vi "ScriptedAutonomous.vi"   [LabVIEW 2015]
uses:
  Common Code/commandCluster.ctl
  Common Code/Change Detect Int.vi
  Robot Global Data.vi
types:
  T1 = typedef "commandCluster.ctl" = cluster{"Step ID":i16, "Command Type":i16, "Drive X":sgl, "Drive Y":sgl, "Heading":sgl, "Max Exec. Time":i16, "Jump Type":i32, "Jump To":i16, "Jump Condition":i16, "Async Drive?":i16, "Roller Mode":i16, "Roller Align":i16, "Roller Closed?":i16, "Wait Condition":i16, "Elevator Mode":i16, "Elevator Command":i16, "Roller State":i16, "Hold Low?":i16, "Num Totes":i16, "Num Cans":dbl, "Past Distance":dbl, "Store Can?":dbl, "X Speed":dbl, "Y Speed":dbl, "Yaw Angle Set":dbl, "Grab Can":dbl, "Roller Overide Speed":dbl, "Force Load?":sgl, "Set Idle":sgl, "Eject":sgl, "Pike Action":sgl, "Pivot Speed":dbl, "Height":dbl}
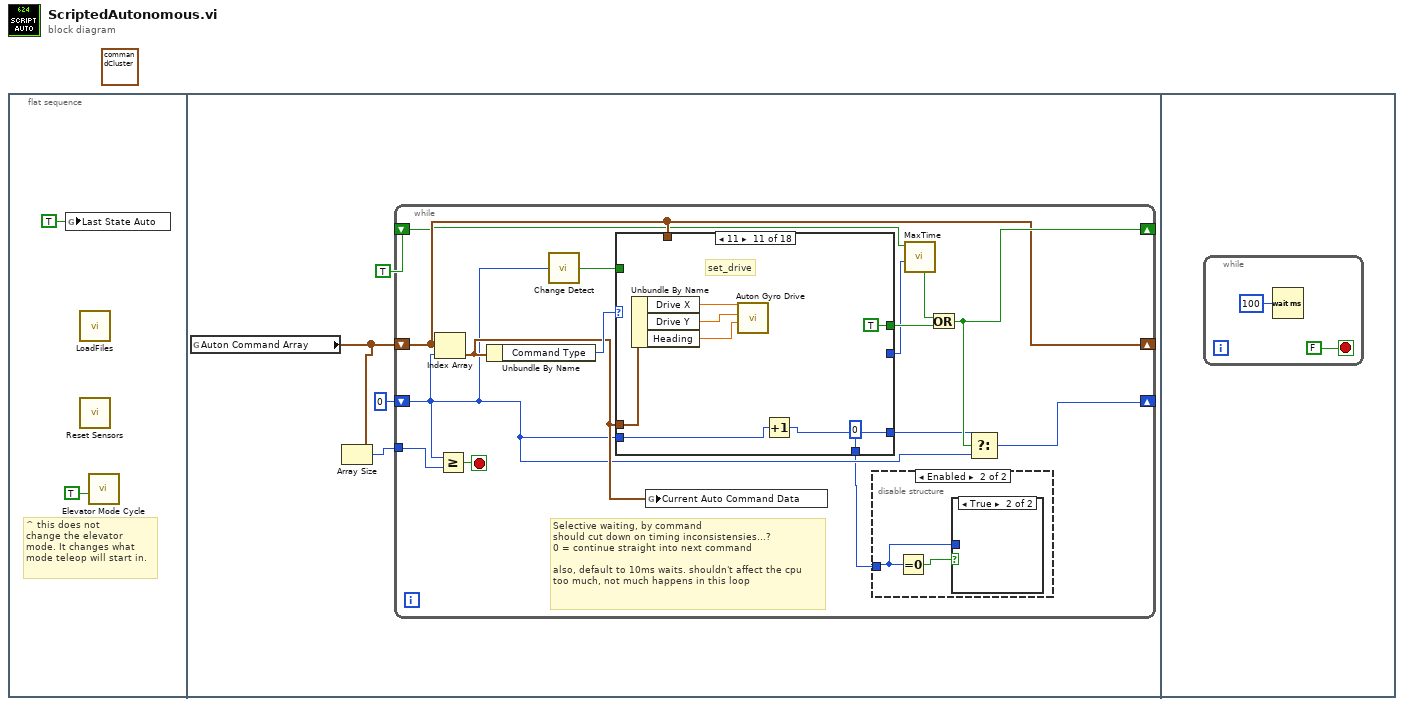
[diagram p0: block diagram]
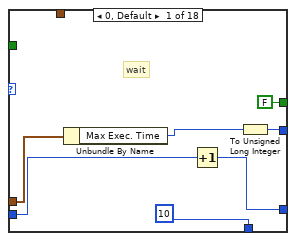
[diagram p2: hidden frame]
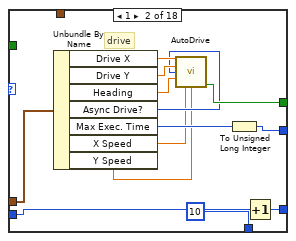
[diagram p3: hidden frame]
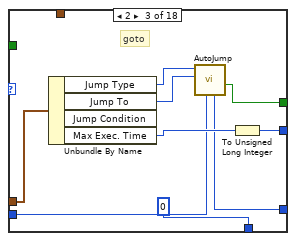
[diagram p4: hidden frame]
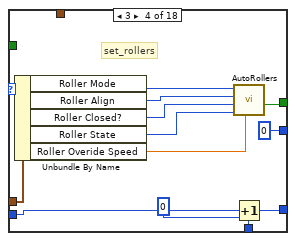
[diagram p5: hidden frame]
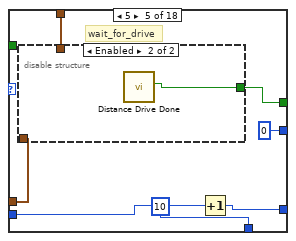
[diagram p6: hidden frame]
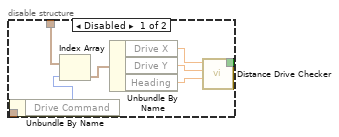
[diagram p7: hidden frame]
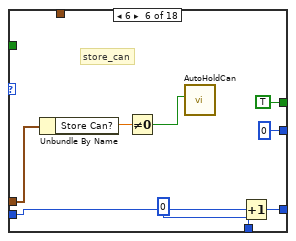
[diagram p8: hidden frame]
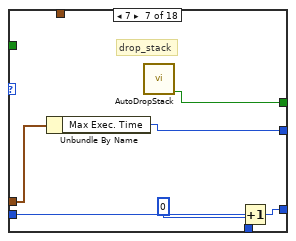
[diagram p9: hidden frame]
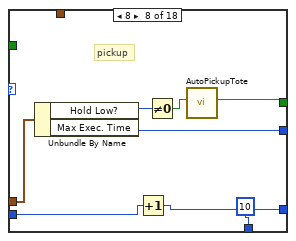
[diagram p10: hidden frame]
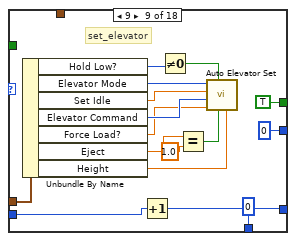
[diagram p11: hidden frame]
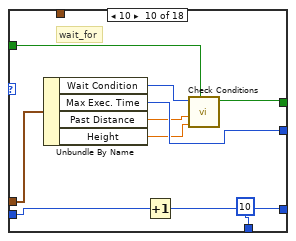
[diagram p12: hidden frame]
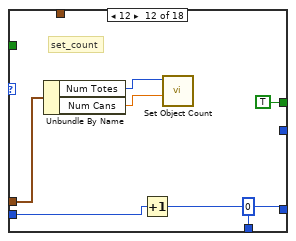
[diagram p13: hidden frame]
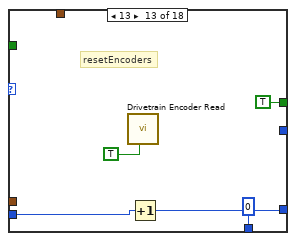
[diagram p14: hidden frame]
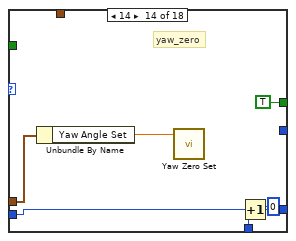
[diagram p15: hidden frame]
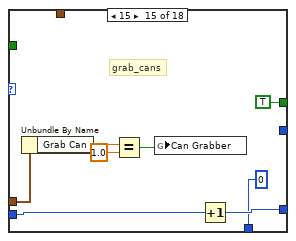
[diagram p16: hidden frame]
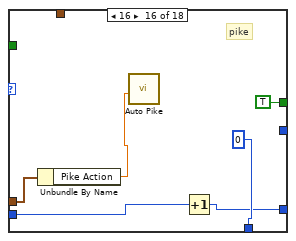
[diagram p17: hidden frame]
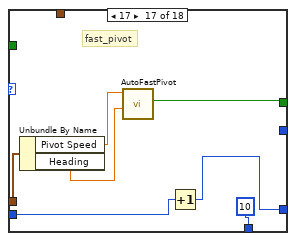
[diagram p18: hidden frame]
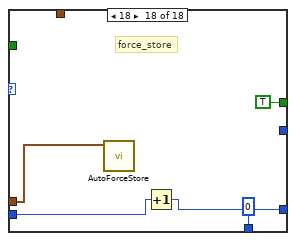
[diagram p19: hidden frame]
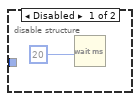
[diagram p20: hidden frame]
diagram:
  (unwired) T1 {"Step ID"=0, "Command Type"=0, "Drive X"=0.0, "Drive Y"=0.0, "Heading"=0.0, "Max Exec. Time"=0, "Jump Type"=0, "Jump To"=0, "Jump Condition"=0, "Async Drive?"=0, "Roller Mode"=0, "Roller Align"=0, "Roller Closed?"=0, "Wait Condition"=0, "Elevator Mode"=0, "Elevator Command"=0, "Roller State"=0, "Hold Low?"=0, "Num Totes"=0, "Num Cans"=0.0, "Past Distance"=0.0, "Store Can?"=0.0, "X Speed"=0.0, "Y Speed"=0.0, "Yaw Angle Set"=0.0, "Grab Can"=0.0, "Roller Overide Speed"=0.0, "Force Load?"=0.0, "Set Idle"=0.0, "Eject"=0.0, "Pike Action"=0.0, "Pivot Speed"=0.0, "Height"=0.0} ("Current Auto Command Data")
  n1 = flat-sequence {
    frame #0 {
      # "^ this does not\nchange the elevator\nmode. It changes what \nmode teleop will start in."
      n2 = global write "Robot Global Data.vi" "Last State Auto"(TRUE ("Last State Auto")) -> ()
      n3 = call "LoadFiles.vi"() -> ()  [unwired: 12 in]
      n4 = call "Reset Sensors.vi"() -> ()  [unwired: 12 in]
      n5 = call "Elevator Mode Cycle.vi"("Set to Auto"=TRUE) -> ()  [unwired: 10 in, 1 out]
    }
    frame #1 {
      n6 = global read "Robot Global Data.vi" "Auton Command Array"() -> (w6:T1[])
      n7 = Array Size(array=w6) -> (size(s)=w3:i32)
      n8 = while {
        shift-right: [w15] -> _
        shift-left: w6 -> [w15]
        shift-right: [w18] -> _
        shift-left: 0 -> [w9]
        shift-right: [w21] -> _
        shift-left: TRUE -> [w10]
        tunnel: w3 -> [w16]
        stop <- w17 stop-if-true
        # "Selective waiting, by command\nshould cut down on timing inconsistensies...?\n0 = continue straight into next command\n\nalso, default to 10ms waits. shouldn't affect the cpu\ntoo much, not much happens in this loop"
        n9 = Index Array(array=w15, index=w9) -> (element=w11:T1)
        n10 = Greater Or Equal?(x=w9, y=w16) -> (x >= y?=w17:bool)
        n11 = Unbundle By Name(w11) -> ("Command Type"=w14:i16)
        n12 = call-poly "Change Detect.vi"("In"=w9) -> ("Changed?"=w8:bool)
        n13 = case shown="11" w14 {
          tunnel: [w25 w39 w50 u32 0 u32 0 u32 0 ("Max Exec. Time") w88 w95 u32 0 ("Max Exec. Time") w121 _ _ _ _ _ _ _ _] -> w13
          tunnel: w11 -> [w28 w30 w48 w61 w66 w81 w91 w96 w106 w122 w133 w140 _ w149 w155 w163 w172 w177]
          tunnel: w9 -> [w27 w41 w43 w60 w65 w83 w90 w98 w115 w125 w128 w136 w144 w150 w158 w160 w167 w176]
          tunnel: [w23 w40 w46 w55 w64 w84 w89 w97 w114 w124 w127 w135 w143 w148 w159 w161 w166 w175] -> w20
          tunnel: [FALSE w38 w47 w59 w67 TRUE ("Done?") w86 w99 TRUE ("Done?") w123 TRUE ("Done?") TRUE ("Done?") TRUE ("Done?") TRUE ("Done?") TRUE ("Done?") TRUE ("Done?") w170 TRUE ("Finished?")] -> w19
          tunnel: w15 -> [_ _ _ _ w68 _ _ _ _ _ _ _ _ _ _ _ _ _]
          tunnel: w8 -> [_ _ _ _ _ _ _ _ _ w118 _ _ _ _ _ _ _ _]
          tunnel: [10 10 0 0 10 0 0 10 0 10 0 0 0 0 0 0 10 0] -> w7
          frame 0, Default {
            # "wait"
            n14 = Unbundle By Name(w28) -> ("Max Exec. Time"=w24:i16)
            n15 = Increment(x=w27) -> (x+1=w23:i32)
            n16 = To Unsigned Long Integer(number=w24) -> (unsigned 32bit integer=w25:u32)
          }
          frame 1 {
            # "drive"
            n17 = Unbundle By Name(w30) -> ("Drive X"=w37:sgl, "Drive Y"=w36:sgl, "Heading"=w35:sgl, "Async Drive?"=w34:i16, "Max Exec. Time"=w33:i16, "X Speed"=w32:dbl, "Y Speed"=w31:dbl)
            n18 = call "AutoDrive.vi"("Drive X"=w37, "Drive Y"=w36, "Async?"=w34, "Heading"=w35, "X Speed"=w32, "Y Speed"=w31) -> ("Done?"=w38:bool)  [unwired: 9 in]
            n19 = To Unsigned Long Integer(number=w33) -> (unsigned 32bit integer=w39:u32)
            n20 = Increment(x=w41) -> (x+1=w40:i32)
          }
          frame 2 {
            # "goto"
            n21 = Unbundle By Name(w48) -> ("Jump Type"=w45:i32, "Jump To"=w44:i16, "Max Exec. Time"=w49:i16)  [unwired: 1 out]
            n22 = call "AutoJump.vi"("Current Index"=w43, "Goto"=w44, "Type"=w45) -> ("Done?"=w47:bool, "New Index"=w46:i32)  [unwired: 7 in]
            n23 = To Unsigned Long Integer(number=w49) -> (unsigned 32bit integer=w50:u32)
          }
          frame 3 {
            # "set_rollers"
            n24 = Unbundle By Name(w61) -> ("Roller Mode"=w58:i16, "Roller Align"=w57:i16, "Roller Closed?"=w56:i16, "Roller State"=w53:i16, "Roller Overide Speed"=w52:dbl)
            n25 = call "AutoRollers.vi"("Override Speed"=w52, "State"=w53, "Close Rollers"=w56, "Align"=w57, "Mode"=w58) -> ("Done?"=w59:bool)  [unwired: 6 in]
            n26 = Increment(x=w60) -> (x+1=w55:i32)
          }
          frame 5 {
            # "wait_for_drive"
            n27 = disable-structure shown="Enabled" {
              disable-tunnel: w68 -> [w76 _]
              disable-tunnel: [w75 w77] -> w67
              disable-tunnel: w66 -> [w69 _]
              frame Disabled {
                n28 = Unbundle By Name(w69) -> ("Drive Command"=w70:i16)
                n29 = Index Array(array=w76, index=w70) -> (element=w71:T1)
                n30 = Unbundle By Name(w71) -> ("Drive X"=w74:sgl, "Drive Y"=w73:sgl, "Heading"=w72:sgl)
                n31 = call "Distance Drive Checker.vi"("Current Heading Target"=w72, "Current Y Target"=w73, "Current X Target"=w74) -> ("Distance Drive Done?"=w75:bool)  [unwired: 8 in]
              }
              frame Enabled {
                n32 = call "Distance Drive Done"() -> ("Done?"=w77:bool)  [unwired: 11 in]
              }
            }
            n33 = Increment(x=w65) -> (x+1=w64:i32)
          }
          frame 6 {
            # "store_can"
            n34 = Unbundle By Name(w81) -> ("Store Can?"=w80:dbl)
            n35 = Not Equal To 0?(x=w80) -> (x != 0?=w79:bool)
            n36 = call "AutoHoldCan.vi"("Store Trashcan?"=w79) -> ()  [unwired: 11 in]
            n37 = Increment(x=w83) -> (x+1=w84:i32)
          }
          frame 7 {
            # "drop_stack"
            n38 = Unbundle By Name(w91) -> ("Max Exec. Time"=w88:i16)
            n39 = call "AutoDropStack.vi"() -> ("Done?"=w86:bool)  [unwired: 11 in]
            n40 = Increment(x=w90) -> (x+1=w89:i32)
          }
          frame 8 {
            # "pickup"
            n41 = Unbundle By Name(w96) -> ("Hold Low?"=w93:i16, "Max Exec. Time"=w95:i16)
            n42 = Increment(x=w98) -> (x+1=w97:i32)
            n43 = Not Equal To 0?(x=w93) -> (x != 0?=w94:bool)
            n44 = call "AutoPickupTote.vi"("Hold Low?"=w94) -> ("Done?"=w99:bool)  [unwired: 10 in]
          }
          frame 9 {
            # "set_elevator"
            n45 = Unbundle By Name(w106) -> ("Hold Low?"=w110:i16, "Elevator Mode"=w109:i16, "Set Idle"=w105:sgl, "Elevator Command"=w108:i16, "Force Load?"=w107:sgl, "Eject"=w103:sgl, "Height"=w100:dbl)
            n46 = Increment(x=w115) -> (x+1=w114:i32)
            n47 = Not Equal To 0?(x=w110) -> (x != 0?=w112:bool)
            n48 = Equal?(x=w103, y=sgl 1.0) -> (x = y?=w101:bool)
            n49 = call "Auto Elevator Set.vi"("Raw Height Set"=w100, "Manual Eject Piston"=w101, "Hold Low"=w112, "Force?"=w107, "Command"=w108, "Set Idle State"=w105, "Mode"=w109) -> ()  [unwired: 5 in]
          }
          frame 10 {
            # "wait_for"
            n50 = Unbundle By Name(w122) -> ("Wait Condition"=w120:i16, "Max Exec. Time"=w121:i16, "Past Distance"=w119:dbl, "Height"=w116:dbl)
            n51 = Increment(x=w125) -> (x+1=w124:i32)
            n52 = call "Check Conditions.vi"("Reset"=w118, "Height"=w116, "Dist"=w119, "Condition"=w120) -> ("Done?"=w123:bool)  [unwired: 7 in]
          }
          frame 11 {
            # "set_drive"
            n53 = Unbundle By Name(w133) -> ("Drive X"=w132:sgl, "Drive Y"=w131:sgl, "Heading"=w130:sgl)
            n54 = call "Auton Gyro Drive.vi"("Heading target"=w130, "Y Speed"=w131, "X Speed"=w132) -> ()  [unwired: 9 in]
            n55 = Increment(x=w128) -> (x+1=w127:i32)
          }
          frame 12 {
            # "set_count"
            n56 = Unbundle By Name(w140) -> ("Num Totes"=w139:i16, "Num Cans"=w138:dbl)
            n57 = Increment(x=w136) -> (x+1=w135:i32)
            n58 = call "Set Object Count.vi"("Num Cans"=w138, "Num Totes"=w139) -> ()  [unwired: 10 in]
          }
          frame 13 {
            # "resetEncoders"
            n59 = call "Drivetrain Encoder Read.vi"("Reset?"=TRUE) -> ()  [unwired: 10 in, 1 out]
            n60 = Increment(x=w144) -> (x+1=w143:i32)
          }
          frame 14 {
            # "yaw_zero"
            n61 = Unbundle By Name(w149) -> ("Yaw Angle Set"=w147:dbl)
            n62 = call "Yaw Zero Set.vi"("Set Angle"=w147) -> ()  [unwired: 11 in]
            n63 = Increment(x=w150) -> (x+1=w148:i32)
          }
          frame 15 {
            # "grab_cans"
            n64 = Unbundle By Name(w155) -> ("Grab Can"=w156:dbl)
            n65 = Equal?(x=w156, y=1.0) -> (x = y?=w154:bool)
            n66 = global write "Robot Global Data.vi" "Can Grabber"(w154) -> ()
            n67 = Increment(x=w158) -> (x+1=w159:i32)
          }
          frame 16 {
            # "pike"
            n68 = Unbundle By Name(w163) -> ("Pike Action"=w162:sgl)
            n69 = call "Auto Pike.vi"("Pike Command"=w162) -> ()  [unwired: 11 in]
            n70 = Increment(x=w160) -> (x+1=w161:i32)
          }
          frame 17 {
            # "fast_pivot"
            n71 = Unbundle By Name(w172) -> ("Pivot Speed"=w168:dbl, "Heading"=w171:sgl)
            n72 = call "AutoFastPivot.vi"("Heading"=w171, "Pivot Speed"=w168) -> ("Finished?"=w170:bool)  [unwired: 9 in]
            n73 = Increment(x=w167) -> (x+1=w166:i32)
          }
          frame 18 {
            # "force_store"
            n74 = call "AutoForceStore.vi"("Command Cluster"=w177) -> ()  [unwired: 11 in]
            n75 = Increment(x=w176) -> (x+1=w175:i32)
          }
        }
        n76 = global write "Robot Global Data.vi" "Current Auto Command Data"(w11) -> ()
        n77 = disable-structure shown="Enabled" {
          disable-tunnel: w7 -> [_ w179]
          frame Disabled {
            n78 = Wait (ms)(milliseconds to wait=u32 20) -> ()  [unwired: 1 out]
          }
          frame Enabled {
            n79 = Equal To 0?(x=w179) -> (x = 0?=w180:bool)
            n80 = case shown="True" w180 {
              tunnel: w179 -> [w181 _]
              frame False {
                n81 = Wait (ms)(milliseconds to wait=w181) -> ()  [unwired: 1 out]
              }
              frame True {
              }
            }
          }
        }
        n82 = call "MaxTime.vi"("maxTime"=w13, "Reset?"=w10) -> ("Finished?"=w12:bool)  [unwired: 9 in]
        n83 = Or(x=w12, y=w19) -> (x .or. y?=w21:bool)
        n84 = Select(t=w20, s=w21, f=w9) -> (s? t:f=w18:i32)
      }
    }
    frame #2 {
      n85 = while {
        stop <- FALSE stop-if-true
        n86 = Wait (ms)(milliseconds to wait=u32 100) -> ()  [unwired: 1 out]
      }
    }
  }
